vi "Processing Loop.vi"(8 "error in (no error)":errorcluster) -> (0 "error out":errorcluster)   [LabVIEW 2017]
uses:
  DEF-SineSettings.ctl
  2051bc23-d823-4102-b9df-3c4968bbf2bf.vi
  5cdb161c-fa3d-464e-9dc8-a8ec64172e4a.vi
  a18540e0-282e-4c56-9306-db85f231deed.vi
  TagDB/_Support/DataAccess/_NameCacher.vi
  TagDB/_Support/DataAccess/_datatypeChecker.vi
  TagDB/_Support/DataAccess/TagDB Ref to DVR.vi
  <vilib>/Utility/error.llb/Trim Whitespace.vi
  TagDB/_Support/Error/_[error50002]Invalid DataType.vi
  TagDB/_Support/Error/_[error50000]Invalid DB REF.vi
  <vilib>/Utility/Data Type/Get Type Information.vi
  <vilib>/measure/NI_MABase.lvlib
  TagDB/TagDB(DEV).lvlib
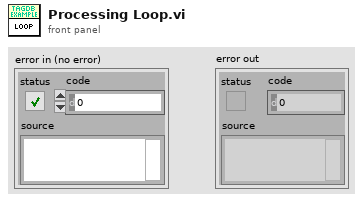
[diagram p1: front panel]
types:
  T1 = typedef "TagDB(DEV).lvlib/TagContainer.ctl" = refnum<k1>
  T2 = typedef "DEF-SineSettings.ctl" = cluster{"frequency":dbl, "amplitude":dbl, "phase":dbl, "sampling info":cluster{"Fs":dbl, "#s":dbl}}
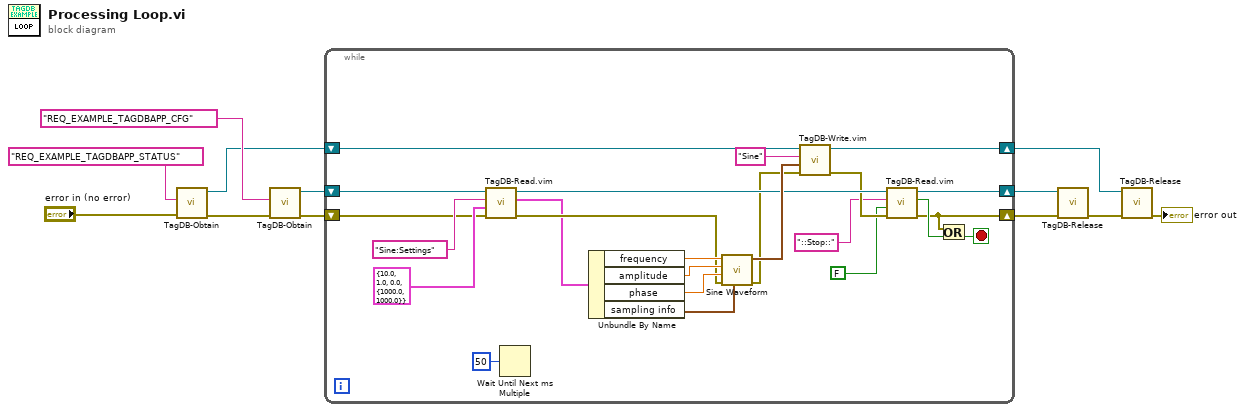
[diagram p0: block diagram]
diagram:
  n1 = call "TagDB-Obtain.vi"("error in (no error)"="error in (no error)", "name (unnamed)"="REQ_EXAMPLE_TAGDBAPP_STATUS") -> ("error out"=w10:errorcluster, "TagContainer"=w6:T1)  [unwired: 3 in, 1 out]
  n2 = call "TagDB-Obtain.vi"("error in (no error)"=w10, "name (unnamed)"="REQ_EXAMPLE_TAGDBAPP_CFG") -> ("error out"=w9:errorcluster, "TagContainer"=w7:T1)  [unwired: 3 in, 1 out]
  n3 = while {
    shift-right: [w17] -> w4
    shift-left: w9 -> [w29]
    shift-right: [w21] -> w3
    shift-left: w7 -> [w28]
    shift-right: [w24] -> w2
    shift-left: w6 -> [w27]
    stop <- w18 stop-if-true
    n4 = call "TagDB-Read.vim"("error in (no error)"=w29, "Type"=T2 {"frequency"=10.0, "amplitude"=1.0, "phase"=0.0, "sampling info"={"Fs"=1000.0, "#s"=1000.0}} ("Sine Settings"), "name"="Sine:Settings", "TagContainer"=w28) -> ("error out"=w16:errorcluster, "Value"=w13:T2, "TagContainer(dup)"=w23:T1)  [unwired: 2 in, 3 out]
    n5 = Wait Until Next ms Multiple(millisecond multiple=u32 50 ("milliseconds to wait")) -> ()  [unwired: 1 out]
    n6 = Unbundle By Name(w13) -> ("frequency"=w33:dbl, "amplitude"=w32:dbl, "phase"=w31:dbl, "sampling info"=w30:cluster{"Fs":dbl, "#s":dbl})
    n7 = call <vilib>:"Sine Waveform.vi"("sampling info"=w30, "error in (no error)"=w16, "phase"=w31, "amplitude"=w32, "frequency"=w33) -> ("error out"=w15:errorcluster, "signal out"=w26:waveform(dbl))  [unwired: 5 in]
    n8 = call "TagDB-Write.vim"("error in (no error)"=w15, "Value"=w26, "name"="Sine", "TagContainer"=w27) -> ("error out"=w22:errorcluster, "TagContainer(dup)"=w24:T1)  [unwired: 5 in, 1 out]
    n9 = call "TagDB-Read.vim"("error in (no error)"=w22, "Type"=FALSE ("Add wih NonExist?"), "name"="::Stop::", "TagContainer"=w23) -> ("error out"=w17:errorcluster, "Value"=w19:bool, "TagContainer(dup)"=w21:T1)  [unwired: 2 in, 3 out]
    n10 = Or(x=w17, y=w19) -> (x .or. y?=w18:bool)
  }
  n11 = call "TagDB-Release.vi"("error in (no error)"=w4, "TagContainer"=w3) -> ("error out"=w5:errorcluster)  [unwired: 9 in]
  n12 = call "TagDB-Release.vi"("error in (no error)"=w5, "TagContainer"=w2) -> ("error out"=→"error out":errorcluster)  [unwired: 9 in]
